vi "Example Set Flowrate.vi"() -> ()   [LabVIEW 2017]
uses:
  <instrlib>/Roboteq Controller KBL1xxx/Roboteq Controller KBL1xxx.lvlib
  Pump Controller.lvlib
panel:
  in  "Pump Flowrate, m^3/s":dbl
  in  "Pump Controller VISA resource name":refnum<visa-resource-name>
  # "TODO: Set Flowrate to Pump Speed Conversion Coefficient in \"Set Flowrate.vi\""
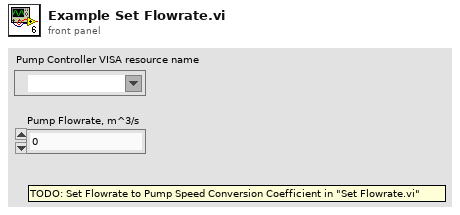
[diagram p1: front panel]
types:
  T1 = typedef "Roboteq Controller KBL1xxx.lvlib/Controller.ctl" = cluster{"VISA resource name out":refnum<visa-resource-name>, "MXRPM":u16}
  T2 = typedef "Pump Controller.lvlib/Pump.ctl" = cluster{"Controller":T1}
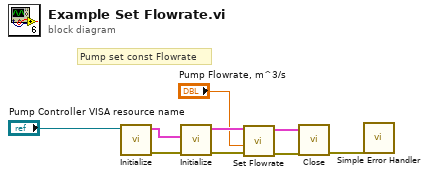
[diagram p0: block diagram]
diagram:
  # "Pump set const Flowrate"
  n1 = call <instrlib>:"Initialize.vi"("VISA resource name"="Pump Controller VISA resource name") -> ("error out"=w7:errorcluster, "Controller"=w8:T1)  [unwired: 9 in]
  n2 = call <instrlib>:"Initialize.vi"("error in (no error)"=w7, "Controller"=w8) -> ("error out"=w6:errorcluster, "Pump"=w5:T2)  [unwired: 8 in]
  n3 = call "Set Flowrate.vi"("error in (no error)"=w6, "Flowrate, m^3/s"="Pump Flowrate, m^3/s", "Pump in"=w5) -> ("error out"=w3:errorcluster, "Pump out"=w2:T2)  [unwired: 7 in]
  n4 = call "Close.vi"("error in (no error)"=w3, "Pump in"=w2) -> ("error out"=w1:errorcluster)  [unwired: 9 in]
  n5 = call <vilib>:"Simple Error Handler.vi"("error in (no error)"=w1) -> ()  [unwired: 4 in, 5 out]
